vi "GetMaxFreqRatio.vi"(8 "错误输入（无错误）":errorcluster, 9 "数据传输模式":u8) -> (0 "错误输出":errorcluster, 3 "返回值":u16)   [LabVIEW 2014]
uses:
  X86Dll/ZXUTConfigMgr.dll
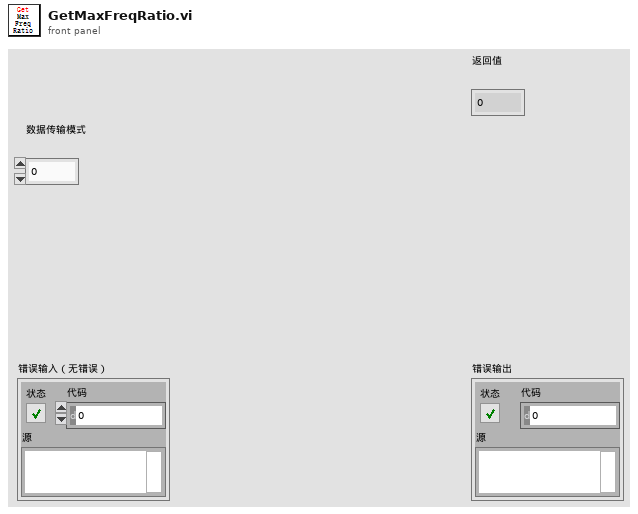
[diagram p1: front panel]
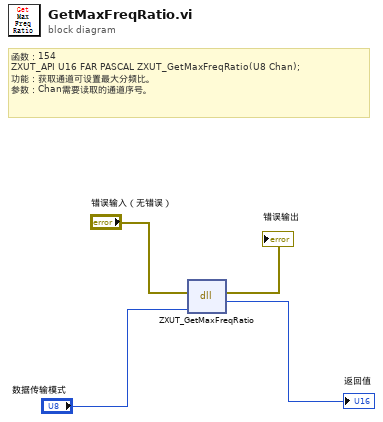
[diagram p0: block diagram]
diagram:
  # "函数：154\nZXUT_API U16\tFAR PASCAL ZXUT_GetMaxFreqRatio(U8 Chan);\n功能：获取通道可设置最大分频比。\n参数：Chan需要读取的通道序号。"
  n1 = dll-call lib="D:/Software/Utrasonic on-line monitoring/X86Dll/ZXUTConfigMgr.dll" fn="ZXUT_GetMaxFreqRatio"(error in="错误输入（无错误）", "Chan"="数据传输模式") -> (error out=→"错误输出":errorcluster, "返回值"=→"返回值":u16)  [unwired: 3 in, 1 out]
